vi "CMN_GetArg.vi"(9 "arg number":u8=1 min=1, 10 "arguments":string) -> (2 "argument":string)   [LabVIEW 2016]
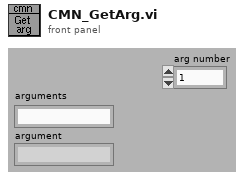
[diagram p1: front panel]
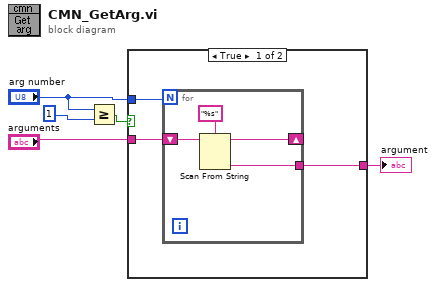
[diagram p0: block diagram]
diagram:
  n1 = Greater Or Equal?(x="arg number", y=1) -> (x >= y?=w1:bool)
  n2 = case shown="True" w1 {
    tunnel: "arguments" -> [w8 w13]
    tunnel: "arg number" -> [w7 _]
    tunnel: [w6 w13] -> w4
    frame True {
      n3 = for {
        N: w7 -> [_]
        shift-right: [w10] -> _
        shift-left: w8 -> [w12]
        tunnel: [w9] -> w6
        n4 = Scan From String(format string="%s", input string=w12) -> (remaining string=w10:string, output 1=w9:string)  [unwired: 2 in, 3 out]
      }
    }
    frame False {
    }
  }
  "argument" <- w4
